vi "Eval y=f(x)_core(VI).vi"(4 "sign":i32(ring) items=["y=f(x)", "y=-f(x)"], 6 "data":variant, 7 "f(x)":T1, 8 "error in":i32, 9 "end":dbl=1.0 format="%.2f", 10 "start":dbl format="%.2f", 11 "number of points":u32=10) -> (0 "error out":i32, 1 "ticks":u32, 2 "Y Values":dbl[](array[numeric]) format="%.2f", 3 "X Values":dbl[](array[numeric]) format="%.2f")   [LabVIEW 2020, in "NI_Gmath.lvlib"]
uses:
  NI_Gmath.lvlib
  functionRefnum.ctl
  Ramp Pattern by Samples.vi
  NI_AALBase.lvlib
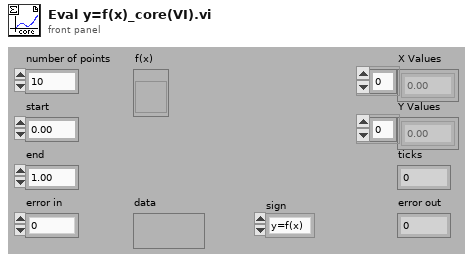
[diagram p1: front panel]
types:
  T1 = typedef "NI_Gmath.lvlib/functionRefnum.ctl" = refnum<vi>
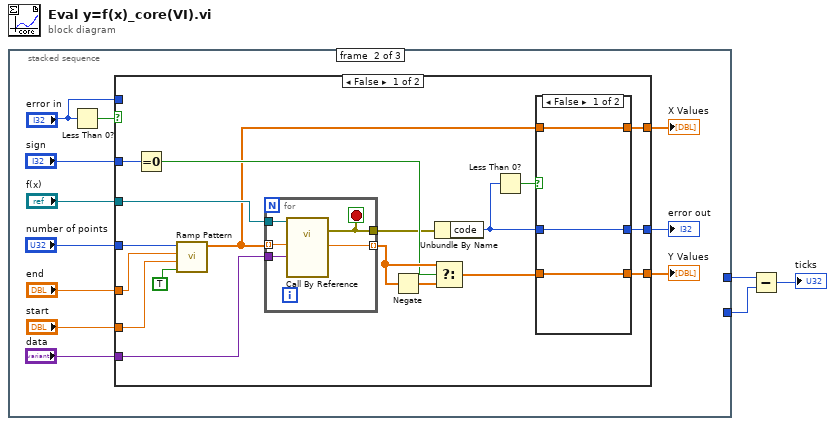
[diagram p0: block diagram]
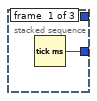
[diagram p2: hidden frame]
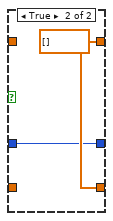
[diagram p3: hidden frame]
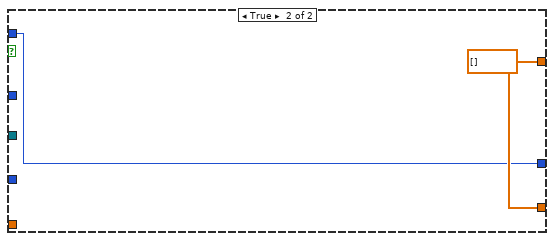
[diagram p4: hidden frame]
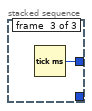
[diagram p5: hidden frame]
diagram:
  n1 = stacked-sequence {
    tunnel: [w4 _ _] -> w2
    tunnel: [_ _ w46] -> w3
    frame #0 {
      n2 = Tick Count (ms)() -> (millisecond timer value=w4:u32)
    }
    frame #1 {
      n3 = Less Than 0?(x="error in") -> (x < 0?=w15:bool)
      n4 = case shown="False" w15 {
        tunnel: [w16 w45] -> w6
        tunnel: [w20 w45] -> w5
        tunnel: "error in" -> [_ w44]
        tunnel: "number of points" -> [w32 _]
        tunnel: "end" -> [w31 _]
        tunnel: "start" -> [w30 _]
        tunnel: "f(x)" -> [w29 _]
        tunnel: "data" -> [w28 _]
        tunnel: "sign" -> [w27 _]
        tunnel: [w19 w44] -> w7
        frame False {
          n5 = Equal To 0?(x=w27) -> (x = 0?=w24:bool)
          n6 = call-poly "Ramp Pattern.vi"("exclude end?"=TRUE, "start"=w30, "end"=w31, "samples"=w32) -> ("Ramp Pattern"=w21:dbl[])  [unwired: 6 in, 1 out]
          n7 = for {
            tunnel: w21 -> [w43] mode=indexing
            tunnel: w28 -> [w42]
            tunnel: w29 -> [w41]
            tunnel: [w40] -> w23
            tunnel: [w39] -> w25 mode=indexing
            stop <- w40 stop-if-true
            n8 = call-by-ref "?"(reference=w41, "Variant"=w42, "x"=w43) -> (error out=w40:errorcluster, "f(x)"=w39:dbl)  [unwired: 4 in, 1 out]
          }
          n9 = Negate(x=w25) -> (-x=w26:dbl[])
          n10 = Select(t=w25, s=w24, f=w26) -> (s? t:f=w17:dbl[])
          n11 = Unbundle By Name(w23) -> ("code"=w18:i32)
          n12 = Less Than 0?(x=w18) -> (x < 0?=w22:bool)
          n13 = case shown="False" w22 {
            tunnel: w17 -> [w36 _]
            tunnel: [w36 w38] -> w16
            tunnel: w21 -> [w35 _]
            tunnel: [w35 w38] -> w20
            tunnel: [w34 w37] -> w19
            tunnel: w18 -> [w34 w37]
            frame False {
            }
            frame True {
              w38 = dbl[] [] ("Ramp Pattern")
            }
          }
        }
        frame True {
          w45 = dbl[] []
        }
      }
      "error out" <- w7
      "X Values" <- w5
      "Y Values" <- w6
    }
    frame #2 {
      n14 = Tick Count (ms)() -> (millisecond timer value=w46:u32)
    }
  }
  n15 = Subtract(x=w3, y=w2) -> (x-y=→"ticks":u32)
